vi "ICR_Setup_Hardware.vi"(8 "error in (no error)":errorcluster, 9 "QMH UI Cluster":variant, 11 "QMH ICR Cluster":T1) -> (0 "error out":errorcluster, 3 "QMH ICR Cluster":T1)   [LabVIEW 2018]
doc: "This VI inits a waveform generation session for both HSDIO 6541 and AWG 5421. This is a basic example that shows how to setup the board in order to generate waveforms according to a script. \n\n1. Initialize for a generation session.\n2. Assign specified channels in Channel List for dynamic operation : all = \"\" (default)\n3. Sets the Idle State for when the generation has completed : NO !!\n4. Configure the Sample clock to use the onboard clock, and configure the clock rate.\n5. Set generation mode to Scripted.\n6. Configure the Script Trigger : change to Digital Edge if waiting for an external\n trigger, and link Rising Edge and source trigger commands.\n Use PFI0 with SMB wired to the board, or any PFIxx if connected to accessory."
uses:
  controls/QMH_ICR_Cluster.ctl
  controls/HARDWARE_Resources.ctl
  controls/PROCESSING_Inputs.ctl
  controls/QMH_UI_Cluster.ctl
  controls/QMH_UI_References.ctl
  controls/QMH_UI_Report.ctl
  controls/QMH_UI_Command.ctl
  controls/QMH_ICR_Command.ctl
  controls/QMH_Status.ctl
  controls/EXPERT_Inputs.ctl
  controls/DIGIT_5122_Inputs.ctl
  <instrlib>/niScope/Controls/niScope trigger source.ctl
  controls/HSDIO_6541_Inputs.ctl
  <instrlib>/niHSDIO/niHSDIO.llb/niHSDIO_ctl Trigger Source Values (Ring).ctl
  controls/SOFTWARE_Inputs.ctl
  controls/AO_6711_Inputs.ctl
  controls/AWG_5421_Inputs.ctl
  <instrlib>/niFgen/niFgen.llb/niFgen_ctl Trigger Source Values (Ring).ctl
  controls/XML_Inputs.ctl
  controls/SEQUENCE_Inputs.ctl
  controls/EXCIT_Inputs.ctl
  controls/DATA_Inputs.ctl
  controls/TIMING_Inputs.ctl
  controls/TRAPPING_Inputs.ctl
panel:
  out "number of samples written per channel":u32 caption="nombre d'échantillons écrits par voie"
  out "Number of Wfms":i32
  out "Script text":string
  out "AWG FIFO used":i64
  out "HSDIO FIFO used":i64
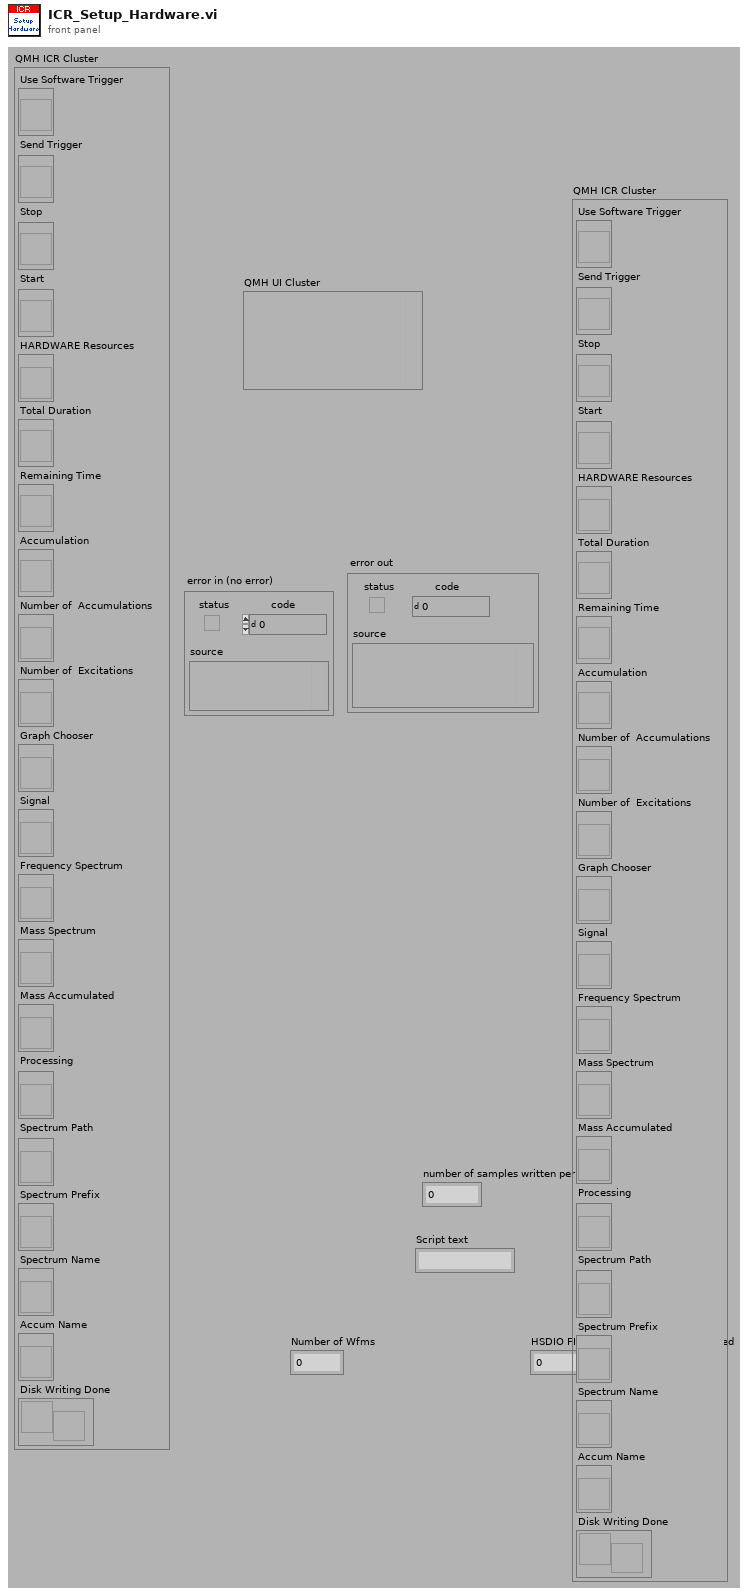
[diagram p1: front panel]
types:
  T1 = typedef "QMH_ICR_Cluster.ctl" = cluster{"Use Software Trigger":refnum<vi>, "Send Trigger":refnum<vi>, "Stop":refnum<vi>, "Start":refnum<vi>, "HARDWARE Resources":refnum<vi>, "Total Duration":refnum<vi>, "Remaining Time":refnum<vi>, "Accumulation":refnum<vi>, "Number of  Accumulations":refnum<vi>, "Number of  Excitations":refnum<vi>, "Graph Chooser":refnum<vi>, "Signal":refnum<vi>, "Frequency Spectrum":refnum<vi>, "Mass Spectrum":refnum<vi>, "Mass Accumulated":refnum<vi>, "Processing":refnum<vi>, "Spectrum Path":refnum<vi>, "Spectrum Prefix":refnum<vi>, "Spectrum Name":refnum<vi>, "Accum Name":refnum<vi>, "Disk Writing Done":refnum<notifier>}
  T2 = typedef "HARDWARE_Resources.ctl" = cluster{"AO6711 Physical Channels":tag, "AO6711 Task Name":refnum<k21>, "AWG5421 Resource Name":refnum<k15>, "DIGIT 5122 Resource Name":refnum<k15>, "HSDIO Resource Name":refnum<k15>}
  T3 = typedef "SEQUENCE_Inputs.ctl" = cluster{"EXCIT Inputs":T4, "DATA Inputs":T5, "TIMING Inputs":T6, "PROCESSING Inputs":T7, "TRAPPING Inputs":T8}
  T4 = typedef "EXCIT_Inputs.ctl" = cluster{"Number of Excitations":i32, "Script Text":string, "Table of Waveforms":string[]}
  T5 = typedef "DATA_Inputs.ctl" = cluster{"Record Length":i32, "Sample Rate":dbl, "Data Type":u8, "Vertical Range":dbl, "Acquisition Duration":dbl}
  T6 = typedef "TIMING_Inputs.ctl" = cluster{"Number of Acquisitions ":i16, "Number of Accumulations":i16, "Table of Waveforms":string[], "Script Text":string}
  T7 = typedef "PROCESSING_Inputs.ctl" = cluster{"Reference Mass":dbl, "Cyclotron Freq":dbl, "Magnetron Freq":dbl}
  T8 = typedef "TRAPPING_Inputs.ctl" = cluster{"Number of Channels":i32, "Init Values":dbl[], "Opening Values":dbl[], "Trapping Values":dbl[], "Emptying Values":dbl[], "Adiabatic ON":bool, "Adiabatic Duration":i32, "Adiabatic Waveforms":string[], "Ions Refill ON":bool, "Number of Ions Refills":i32, "Trapping Delay":dbl, "Trapping Duration":dbl}
  T9 = typedef "EXPERT_Inputs.ctl" = cluster{"DIGIT 5122 Inputs":T10, "HSDIO 6541 Inputs":T12, "SOFTWARE Inputs":T14, "AO 6711 Inputs":T15, "AWG 5421 Inputs":T16, "XML Inputs":T18}
  T10 = typedef "DIGIT_5122_Inputs.ctl" = cluster{"Sample Rate":dbl, "Resource Name":refnum<k15>, "Channel Name":string, "Trigger Source":T11, "Vertical Range":dbl, "Trigger Level":dbl}
  T11 = typedef "niScope trigger source.ctl" = string
  T12 = typedef "HSDIO_6541_Inputs.ctl" = cluster{"Resource Name":refnum<k15>, "Clock Rate":dbl, "Trigger Source":T13}
  T13 = typedef "niHSDIO_ctl Trigger Source Values (Ring).ctl" = string
  T14 = typedef "SOFTWARE_Inputs.ctl" = cluster{"Application Directory":path, "Software Version":string, "Data Path":path, "XML Path":path, "XML File Filter":string, "XML Saved Path":path, "Excit Scripts Path":path, "Excit Scripts File Filter":string, "Excit Waveforms Path":path, "Excit Waveforms File Filter":string, "Timing Scripts Path":path, "Timing Scripts File Filter":string, "Timing Waveforms Path":path, "Timing Waveforms File Filter":string, "Trapping Waveforms Path":path, "Trapping Waveforms File Filter":string}
  T15 = typedef "AO_6711_Inputs.ctl" = cluster{"Physical Channels":tag, "Min Voltage":dbl, "Max Voltage":dbl, "Trigger Source":tag, "Counter":tag}
  T16 = typedef "AWG_5421_Inputs.ctl" = cluster{"Resource Name":refnum<k15>, "Sample Rate":dbl, "Trigger Type":u16, "Trigger Source":T17, "Waveform Gain":dbl, "Digital Filter ON":bool}
  T17 = typedef "niFgen_ctl Trigger Source Values (Ring).ctl" = string
  T18 = typedef "XML_Inputs.ctl" = cluster{"Version Tag Name":string, "Version String":string}
  T19 = typedef "QMH_UI_Cluster.ctl" = cluster{"QMH UI References":T20, "QMH UI Report":T21}
  T20 = typedef "QMH_UI_References.ctl" = cluster{"Refnum Load":refnum<vi>, "Refnum Save As":refnum<vi>, "Refnum Start":refnum<vi>, "Refnum Exit":refnum<vi>, "Refnum Tabs":refnum<vi>, "Refnum SPECTRUM":refnum<vi>, "Refnum EXPERIMENT":refnum<vi>, "Refnum VOLTAGES":refnum<vi>, "Refnum SEQUENCE":refnum<vi>, "Refnum EXPERT":refnum<vi>, "Refnum EXCIT Table":refnum<vi>, "Refnum TIMING Table":refnum<vi>, "Refnum CHANGE Experiment":refnum<vi>, "Refnum CHANGE Voltages":refnum<vi>, "Refnum CHANGE Sequence":refnum<vi>, "Refnum CHANGE Expert":refnum<vi>, "Refnum CHANGE Scientist":refnum<vi>, "Refnum PIL Status":refnum<vi>}
  T21 = typedef "QMH_UI_Report.ctl" = cluster{"UI Status":T22, "ICR Status":T23, "QMH Status":T24}
  T22 = typedef "QMH_UI_Command.ctl" = enum16{"Initialize", "UI Load", "UI Save", "UI Save As", "UI Change Experiment", "UI Change Voltages", "UI Change Sequence", "UI Change Expert", "UI Change Scientist", "Ready to Start", "UI Start", "Waiting for ICR", "UI Exit", "Update Report", "Update ICR Status", "Waiting for User"}
  T23 = typedef "QMH_ICR_Command.ctl" = enum16{"Initialize", "Sequence Setup", "ICR Start", "ICR Stop", "Hardware Setup", "Next Accumulation", "Waiting for Trigger", "Sequence Started", "Sequence Finished", "Writing Data", "Hardware Reset", "Exit"}
  T24 = typedef "QMH_Status.ctl" = enum16{"Init", "Loading", "Setup", "Ready to Start", "Started", "Idle"}
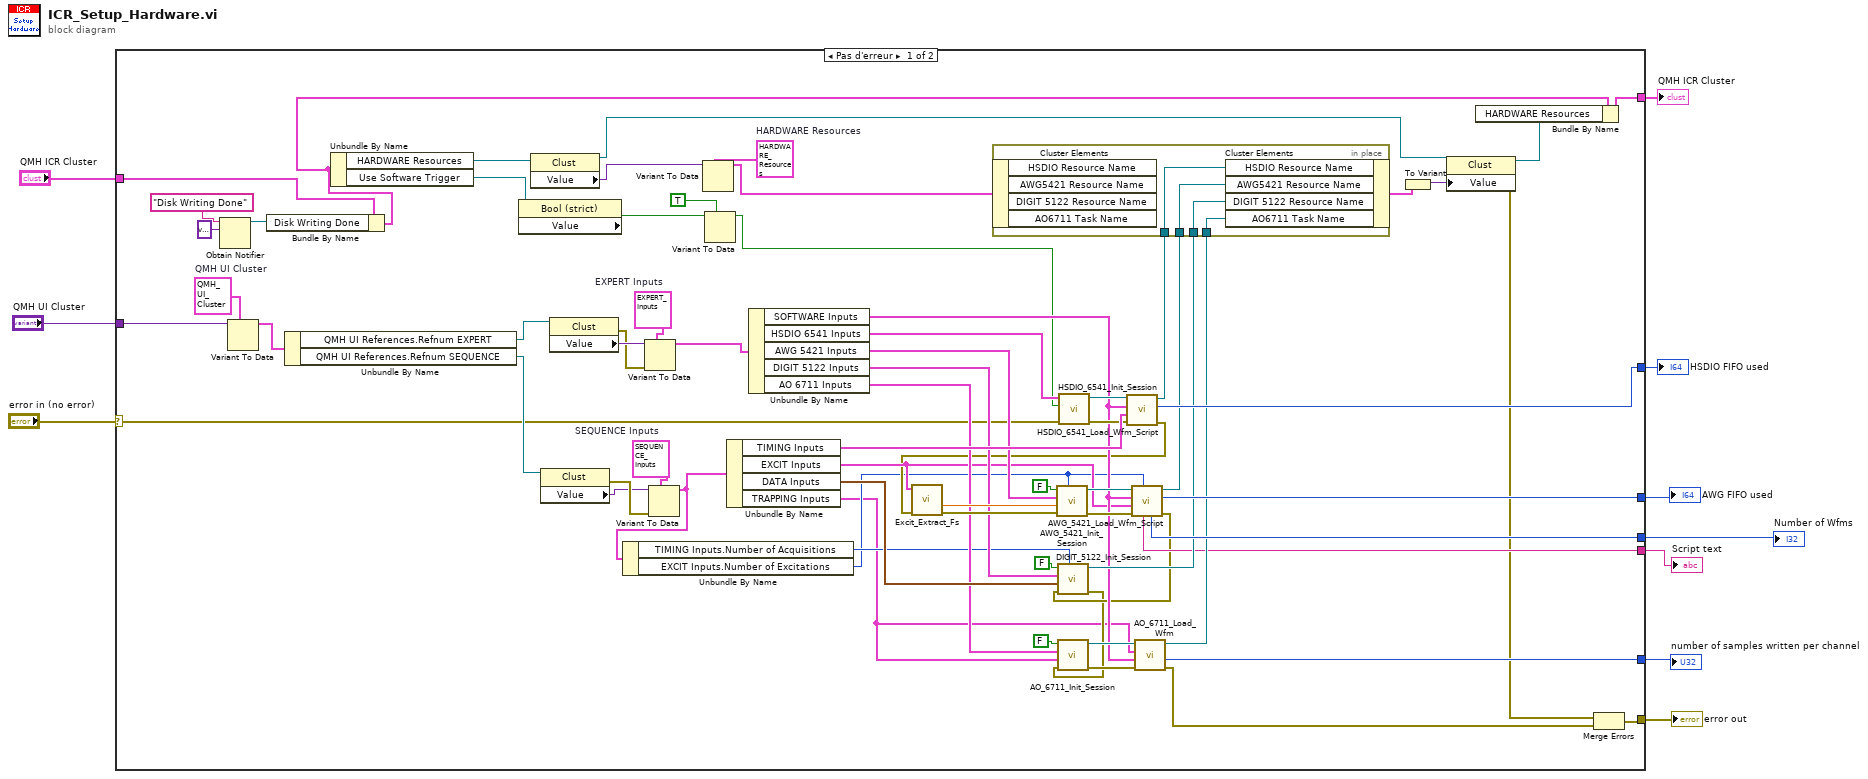
[diagram p0: block diagram]
diagram:
  n1 = case shown="Pas d'erreur" "error in (no error)" {
    selector: "error in (no error)" -> [w16 w85]
    tunnel: [w27 w85] -> w10
    tunnel: "QMH UI Cluster" -> [w79 _]
    tunnel: [w64 _] -> w7
    tunnel: [w60 _] -> w6
    tunnel: [w57 _] -> w4
    tunnel: [w40 _] -> w5
    tunnel: [w42 _] -> w3
    tunnel: "QMH ICR Cluster" -> [w18 w84]
    tunnel: [w23 w84] -> w1
    frame No Error {
      w38 = T2 {"AO6711 Physical Channels"="Analog/ao0:3", "AO6711 Task Name"="", "AWG5421 Resource Name"="Waveform", "DIGIT 5122 Resource Name"="Digitizer", "HSDIO Resource Name"="Sequencer"}  # HARDWARE Resources
      w69 = T3 {"EXCIT Inputs"={"Number of Excitations"=1, "Script Text"="", "Table of Waveforms"=[]}, "DATA Inputs"={"Record Length"=8192, "Sample Rate"=2.0, "Data Type"=1, "Vertical Range"=0.0, "Acquisition Duration"=100000.0}, "TIMING Inputs"={"Number of Acquisitions "=32767, "Number of Accumulations"=1, "Table of Waveforms"=[], "Script Text"=""}, "PROCESSING Inputs"={"Reference Mass"=300.0939, "Cyclotron Freq"=255.727, "Magnetron Freq"=0.001}, "TRAPPING Inputs"={"Number of Channels"=4, "Init Values"=[2.0, 5.0, 5.0, 2.0], "Opening Values"=[0.0, 0.0, 0.0, 0.0], "Trapping Values"=[2.0, 5.0, 5.0, 2.0], "Emptying Values"=[-5.0, -5.0, -5.0, -5.0], "Adiabatic ON"=FALSE, "Adiabatic Duration"=0, "Adiabatic Waveforms"=["Adiabatic_None_2_2_2000.bin", "Adiabatic_Ramp_5_0_2000.bin", "Adiabatic_DoubleRamp_5_0_2000.bin", "Adiabatic_RC_2_0_2000.bin"], "Ions Refill ON"=FALSE, "Number of Ions Refills"=4, "Trapping Delay"=400.0, "Trapping Duration"=300.0}}  # SEQUENCE Inputs
      w74 = T9 {"DIGIT 5122 Inputs"={"Sample Rate"=9.0, "Resource Name"="Digitizer", "Channel Name"="0", "Trigger Source"="VAL_EXTERNAL", "Vertical Range"=10.0, "Trigger Level"=3.0}, "HSDIO 6541 Inputs"={"Resource Name"="SequencerHSDIO", "Clock Rate"=1000000.0, "Trigger Source"="PFI0"}, "SOFTWARE Inputs"={"Application Directory"=path "D:/S.O.F.T.S/LABVIEW/PIL", "Software Version"="1.0.0", "Data Path"=path "D:/PIRENEA/DATA", "XML Path"=path "D:/PIRENEA/DATA", "XML File Filter"="*.xml", "XML Saved Path"=path "D:/PIRENEA/DATA", "Excit Scripts Path"=path "D:/PIRENEA/EXCIT_SCRIPTS", "Excit Scripts File Filter"="*.txt", "Excit Waveforms Path"=path "D:/PIRENEA/EXCIT_WFMS", "Excit Waveforms File Filter"="*.bin", "Timing Scripts Path"=path "D:/PIRENEA/SEQUENCE_SCRIPTS", "Timing Scripts File Filter"="*.txt", "Timing Waveforms Path"=path "D:/PIRENEA/SEQUENCE_WFMS", "Timing Waveforms File Filter"="*.bin", "Trapping Waveforms Path"=path "D:/PIRENEA/TRAPPING_WFMS", "Trapping Waveforms File Filter"="*.bin"}, "AO 6711 Inputs"={"Physical Channels"="AnalogOutput/ao0:3", "Min Voltage"=-10.0, "Max Voltage"=10.0, "Trigger Source"="/AnalogOutput/PFI0", "Counter"="AnalogOutput/ctr0"}, "AWG 5421 Inputs"={"Resource Name"="WaveformGenerator", "Sample Rate"=20000000.0, "Trigger Type"=2, "Trigger Source"="PFI0", "Waveform Gain"=0.31, "Digital Filter ON"=TRUE}, "XML Inputs"={"Version Tag Name"="XML_Version", "Version String"="1.0"}}  # EXPERT Inputs
      w78 = T19 {"QMH UI References"={"Refnum Load"=refnum, "Refnum Save As"=refnum, "Refnum Start"=refnum, "Refnum Exit"=refnum, "Refnum Tabs"=refnum, "Refnum SPECTRUM"=refnum, "Refnum EXPERIMENT"=refnum, "Refnum VOLTAGES"=refnum, "Refnum SEQUENCE"=refnum, "Refnum EXPERT"=refnum, "Refnum EXCIT Table"=refnum, "Refnum TIMING Table"=refnum, "Refnum CHANGE Experiment"=refnum, "Refnum CHANGE Voltages"=refnum, "Refnum CHANGE Sequence"=refnum, "Refnum CHANGE Expert"=refnum, "Refnum CHANGE Scientist"=refnum, "Refnum PIL Status"=refnum}, "QMH UI Report"={"UI Status"=enum."Initialize", "ICR Status"=enum."Initialize", "QMH Status"=enum."Init"}}  # QMH UI Cluster
      n2 = Obtain Notifier(name (unnamed)="Disk Writing Done" ("nom (aucun)"), notification data type=variant ("type de l'élément")) -> (notifier out=w20:refnum<notifier>)  [unwired: 2 in, 2 out]
      n3 = Variant To Data(type=w78, Variant=w79) -> (data=w77:T19)  [unwired: 1 in, 1 out]
      n4 = Bundle By Name(cluster=w18, "Disk Writing Done"=w20) -> (w17:T1)
      n5 = Unbundle By Name(w77) -> ("QMH UI References.Refnum EXPERT"=w76:refnum<vi>, "QMH UI References.Refnum SEQUENCE"=w67:refnum<vi>)
      n6 = Unbundle By Name(w17) -> ("HARDWARE Resources"=w30:refnum<vi>, "Use Software Trigger"=w29:refnum<vi>)
      n7 = property class="Bool (strict)"(reference=w29) -> ("Value"=w35:bool)  [unwired: 1 in, 2 out]
      n8 = property class="Clust"(reference=w30) -> (reference out=w32:refnum<vi>, "Value"=w36:variant)  [unwired: 1 in, 1 out]
      n9 = property class="Clust"(reference=w67) -> (error out=w70:errorcluster, "Value"=w68:variant)  [unwired: 1 in, 1 out]
      n10 = property class="Clust"(reference=w76) -> (error out=w71:errorcluster, "Value"=w75:variant)  [unwired: 1 in, 1 out]
      n11 = Variant To Data(error in=w71, type=w74, Variant=w75) -> (data=w73:T9)  [unwired: 1 out]
      n12 = Variant To Data(error in=w70, type=w69, Variant=w68) -> (data=w26:T3)  [unwired: 1 out]
      n13 = Unbundle By Name(w26) -> ("TIMING Inputs.Number of Acquisitions"=w25:i16, "EXCIT Inputs.Number of Excitations"=w12:i32)
      n14 = Variant To Data(type=w38, Variant=w36) -> (data=w37:T2)  [unwired: 1 in, 1 out]
      n15 = Variant To Data(type=TRUE, Variant=w35) -> (data=w33:bool)  [unwired: 1 in, 1 out]
      n16 = Unbundle By Name(w26) -> ("TIMING Inputs"=w66:T6, "EXCIT Inputs"=w39:T4, "DATA Inputs"=w51:T5, "TRAPPING Inputs"=w11:T8)
      n17 = Unbundle By Name(w73) -> ("SOFTWARE Inputs"=w45:T14, "HSDIO 6541 Inputs"=w72:T12, "AWG 5421 Inputs"=w55:T16, "DIGIT 5122 Inputs"=w52:T10, "AO 6711 Inputs"=w48:T15)
      n18 = call "HSDIO_6541_Init_Session.vi"("error in (no error)"=w16, "Use Software Trigger"=w33, "HSDIO 6541 Inputs"=w72) -> ("error out"=w59:errorcluster, "instrument handle out"=w58:refnum<k15>)  [unwired: 7 in]
      n19 = call "HSDIO_6541_Load_Wfm_Script.vi"("error  in"=w59, "TIMING Inputs"=w66, "SOFTWARE Inputs"=w45, "instrument handle in"=w58) -> ("error out"=w15:errorcluster, "FIFO used"=w64:i64, "instrument handle out"=w65:refnum<k15>)  [unwired: 4 in, 1 out]
      n20 = call "Excit_Extract_Fs.vi"("error in (no error)"=w15, "EXCIT Inputs"=w39) -> ("error out"=w56:errorcluster, "Sample Rate"=w54:dbl)  [unwired: 8 in]
      n21 = call "AWG_5421_Init_Session.vi"("Number of Excitations"=w12, "error in (no error)"=w56, "Sample Rate"=w54, "AWG 5421 Inputs"=w55, "Use Software Trigger"=FALSE) -> ("error out"=w62:errorcluster, "Instrument handle out"=w63:refnum<k15>)  [unwired: 5 in]
      n22 = call "AWG_5421_Load_Wfm_Script.vi"("Number of Excitations"=w12, "error  in"=w62, "EXCIT Inputs"=w39, "SOFTWARE Inputs"=w45, "instrument handle in"=w63) -> ("error out"=w14:errorcluster, "FIFO used"=w60:i64, "instrument handle out"=w61:refnum<k15>, "Number of Wfms"=w57:i32, "Script text"=w40:string)  [unwired: 2 in]
      n23 = call "DIGIT_5122_Init_Session.vi"("Number of Acquisitions"=w25, "error in (no error)"=w14, "DATA Inputs"=w51, "DIGIT 5122 Inputs"=w52, "Use Software Trigger"=FALSE) -> ("error out"=w13:errorcluster, "instrument handle out"=w50:refnum<k15>)  [unwired: 5 in]
      n24 = call "AO_6711_Init_Session.vi"("error in (no error)"=w13, "TRAPPING Inputs"=w11, "AO 6711 Inputs"=w48, "Use Software Trigger"=FALSE) -> ("error out"=w44:errorcluster, "Instrument handle out"=w46:refnum<k21>)  [unwired: 6 in]
      n25 = call "AO_6711_Load_Wfm.vi"("error in (no error)"=w44, "SOFTWARE Inputs"=w45, "TRAPPING Inputs"=w11, "Instrument handle in"=w46) -> ("error out"=w43:errorcluster, "number of samples written per channel"=w42:u32, "Instrument handle out"=w41:refnum<k21>)  [unwired: 4 in, 1 out]
      n26 = in-place {
        in-place-border: w65 -> [w83]
        in-place-border: w61 -> [w82]
        in-place-border: w50 -> [w81]
        in-place-border: w41 -> [w80]
        n27 = in-place-cluster #1(w37) -> ()  [unwired: 4 out]
        n28 = in-place-cluster #1("HSDIO Resource Name"=w83, "AWG5421 Resource Name"=w82, "DIGIT 5122 Resource Name"=w81, "AO6711 Task Name"=w80) -> (w31:T2)
      }
      n29 = To Variant(anything=w31) -> (Variant=w24:variant)
      n30 = property class="Clust"(reference=w32, "Value"=w24) -> (reference out=w22:refnum<vi>, error out=w28:errorcluster)  [unwired: 1 in]
      n31 = Bundle By Name(cluster=w17, "HARDWARE Resources"=w22) -> (w23:T1)
      n32 = Merge Errors(w28, w43) -> (w27:errorcluster)
    }
    frame Error {
    }
  }
  "error out" <- w10
  "HSDIO FIFO used" <- w7
  "AWG FIFO used" <- w6
  "Script text" <- w5
  "Number of Wfms" <- w4
  "number of samples written per channel" <- w3
  "QMH ICR Cluster" <- w1
